vi "optionsAcq_channel_attenuatorState.vi"(6 "poll write":bool, 8 "error in (no error)":errorcluster, 9 "readWrite":enum16{"read", "write"}(ring), 10 "attenFilter_active":bool, 11 "OSAchannel in":refnum<class "OSAchannel.lvclass">) -> (0 "error out":errorcluster, 1 "FTSLib status":i32, 2 "attenFilter_active read":bool, 3 "OSAchannel out":refnum<class "OSAchannel.lvclass">, 4 "poll timeOut":bool)   [LabVIEW 2010, in "OSAchannel.lvclass"]
uses:
  OSAchannel.lvclass
  OSAchannel.lvclass/OSAchannel.ctl
  FTSLib.dll
  OSA20X_misc.lvlib
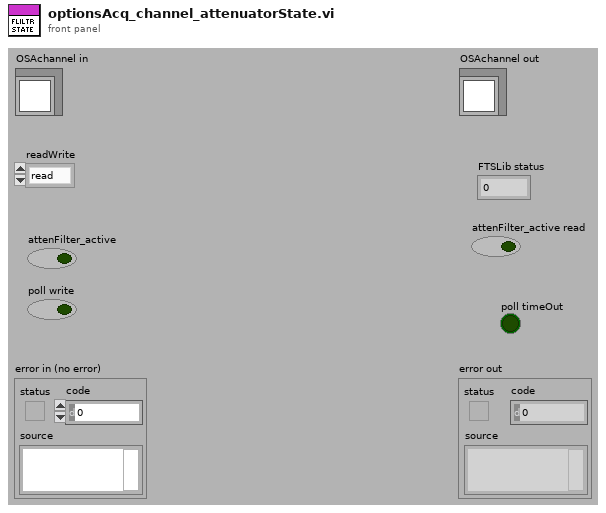
[diagram p1: front panel]
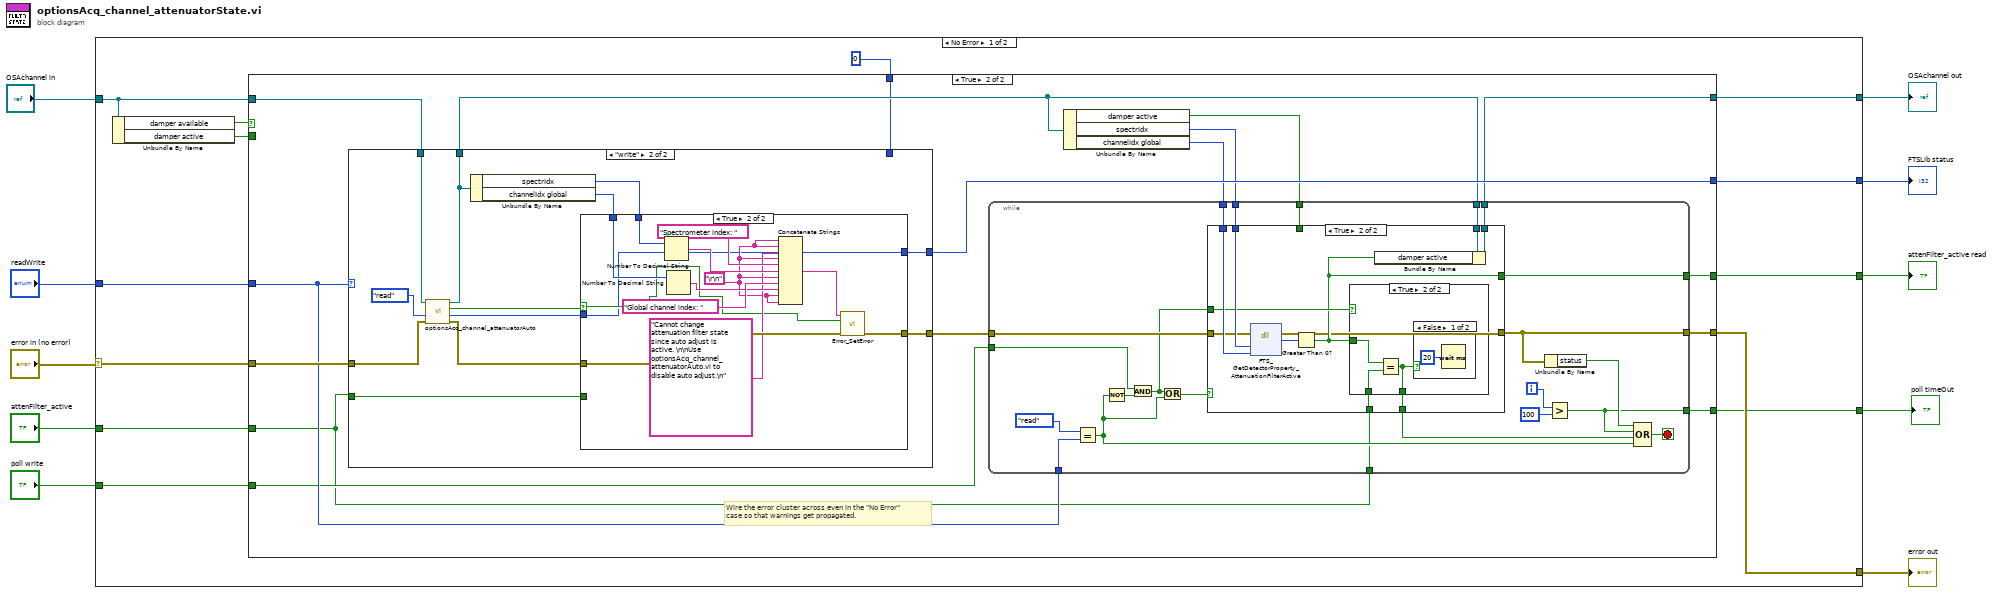
[diagram p0: block diagram]
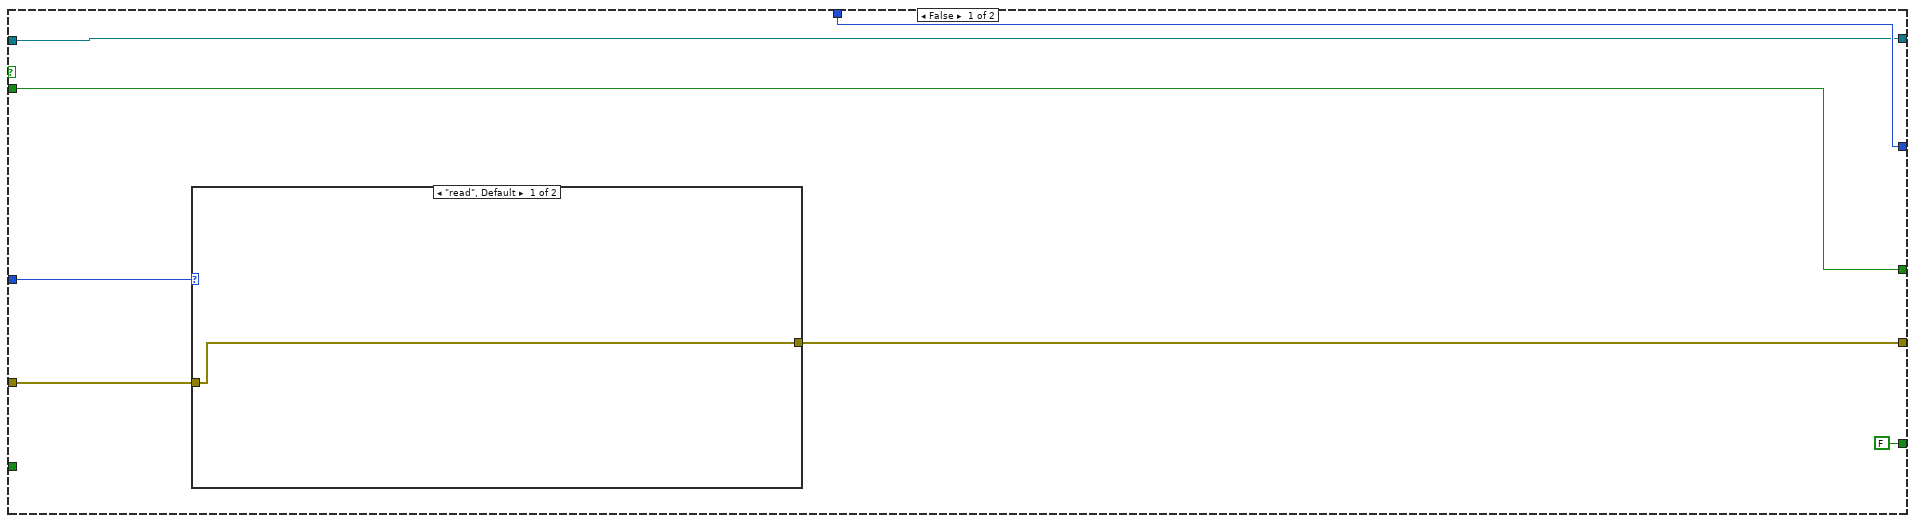
[diagram p2: hidden frame]
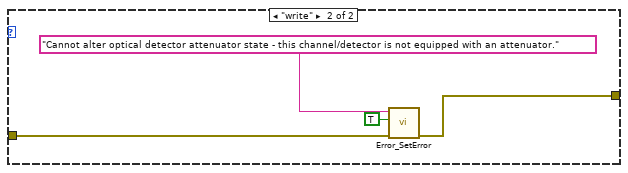
[diagram p3: hidden frame]
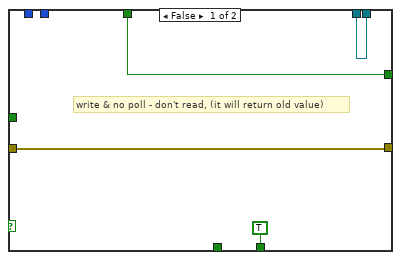
[diagram p4: hidden frame]
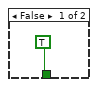
[diagram p5: hidden frame]
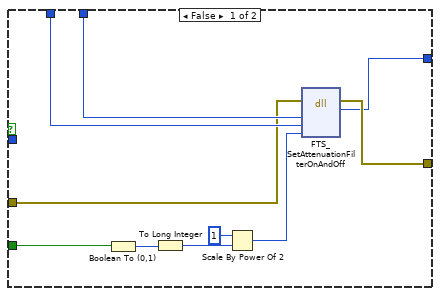
[diagram p8: hidden frame]
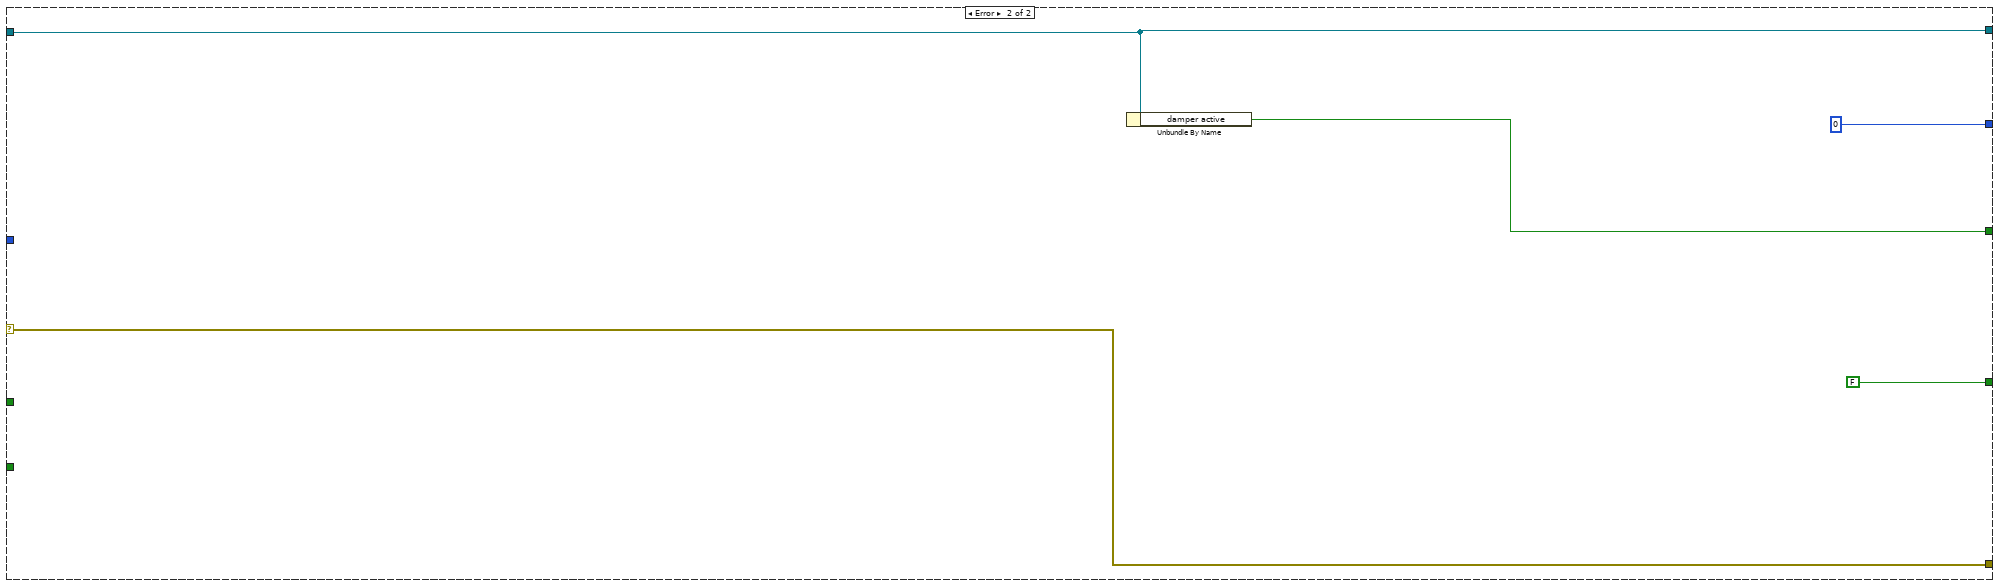
[diagram p9: hidden frame]
diagram:
  n1 = case shown="No Error" "error in (no error)" {
    selector: "error in (no error)" -> [w23 w136]
    tunnel: [w16 w136] -> w9
    tunnel: [w17 w135] -> w7
    tunnel: "OSAchannel in" -> [w14 w135]
    tunnel: "readWrite" -> [w21 _]
    tunnel: "attenFilter_active" -> [w19 _]
    tunnel: [w22 0 ("result")] -> w4
    tunnel: "poll write" -> [w20 _]
    tunnel: [w18 w134] -> w2
    tunnel: [w15 FALSE] -> w1
    frame No Error {
      n2 = Unbundle By Name(w14) -> ("damper available"=w13:bool, "damper active"=w12:bool)
      n3 = case shown="True" w13 {
        tunnel: w23 -> [w25 w51]
        tunnel: [w28 w50] -> w22
        tunnel: w21 -> [w26 w49]
        tunnel: w20 -> [_ w45]
        tunnel: w19 -> [_ w44]
        tunnel: [w30 w43] -> w18
        tunnel: [w27 w42] -> w17
        tunnel: [w24 w40] -> w16
        tunnel: [FALSE w39] -> w15
        tunnel: w14 -> [w27 w37]
        tunnel: w12 -> [w30 _]
        tunnel: 0 ("result") -> [w28 w36]
        frame False {
          n4 = case shown="\"read\", Default" w26 {
            tunnel: w25 -> [w31 w35]
            tunnel: [w31 w34] -> w24
            frame "read", Default {
            }
            frame "write" {
              n5 = call "Error_SetError.vi"("error in"=w35, "status (true)"=TRUE, "source(\"\")"="Cannot alter optical detector attenuator state - this channel/detector is not equipped with an attenuator." ("source(\"\")")) -> ("error out"=w34:errorcluster)  [unwired: 4 in]
            }
          }
        }
        frame True {
          # "Wire the error cluster across even in the \"No Error\"\ncase so that warnings get propagated."
          n6 = case shown="\"write\"" w49 {
            tunnel: [w96 w107] -> w50
            tunnel: w51 -> [w95 w99]
            tunnel: [w95 w108] -> w46
            tunnel: w44 -> [_ w106]
            tunnel: w36 -> [w96 _]
            tunnel: w37 -> [w94 w102]
            tunnel: [w94 w103] -> w38
            frame Default {
            }
            frame "write" {
              n7 = call "optionsAcq_channel_attenuatorAuto.vi"("error in (no error)"=w99, "readWrite"=enum16{"read", "write"}."read", "OSAchannel in"=w102) -> ("error out"=w98:errorcluster, "FTSLib status"=w97:i32, "auto read"=w101:bool, "OSAchannel out"=w103:refnum<class "OSAchannel.lvclass">)  [unwired: 5 in]
              n8 = Unbundle By Name(w103) -> ("spectrIdx"=w104:u16, "channelIdx global"=w105:u16)
              n9 = case shown="True" w101 {
                selector: w101 -> [_ w120]
                tunnel: w105 -> [w118 w128]
                tunnel: w104 -> [w117 w129]
                tunnel: w98 -> [w116 w131]
                tunnel: [w115 w130] -> w108
                tunnel: [w114 w119] -> w107
                tunnel: w106 -> [w109 _]
                tunnel: w97 -> [_ w119]
                frame False {
                  n10 = Boolean To (0,1)(Boolean=w109) -> (0, 1=w111:i16)
                  n11 = To Long Integer(number=w111) -> (32bit integer=w112:i32)
                  n12 = Scale By Power Of 2(n=1, x=w112) -> (x*2^n=w110:i32)
                  n13 = dll-call lib="FTSLib.dll" fn="FTS_SetAttenuationFilterOnAndOff"(error in=w116, "spectrIdx"=w117, "channeldx"=w118, "filterStatus"=w110) -> (error out=w115:errorcluster, "result"=w114:i32)  [unwired: 5 in, 1 out]
                }
                frame True {
                  w121 = "\r\n"
                  n14 = Number To Decimal String(number=w129) -> (decimal integer string=w126:string)  [unwired: 1 in]
                  n15 = Number To Decimal String(number=w128) -> (decimal integer string=w124:string)  [unwired: 1 in]
                  n16 = Concatenate Strings(w121, w121, "Cannot change attenuation filter state since auto adjust is active. \n\nUse optionsAcq_channel_attenuatorAuto.vi to disable auto adjust.\n" ("source(\"\")"), w121, "Spectrometer index: " ("string"), w126, w121, "Global channel index: " ("string"), w124, w121, w121) -> (w122:string)
                  n17 = call "Error_SetError.vi"("error in"=w131, "status (true)"=w120, "source(\"\")"=w122) -> ("error out"=w130:errorcluster)  [unwired: 4 in]
                }
              }
            }
          }
          n18 = Unbundle By Name(w38) -> ("damper active"=w41:bool, "spectrIdx"=w47:u16, "channelIdx global"=w48:u16)
          n19 = while {
            tunnel: w49 -> [w73]
            tunnel: w48 -> [w70]
            tunnel: w47 -> [w69]
            tunnel: w46 -> [w68]
            tunnel: w45 -> [w64]
            tunnel: w44 -> [w63]
            tunnel: [w60] -> w43
            tunnel: w38 -> [w59]
            tunnel: [w58] -> w42
            tunnel: w41 -> [w57]
            tunnel: [w53] -> w40
            tunnel: [w52] -> w39
            i -> [w56]
            stop <- w71 stop-if-true
            n20 = Equal?(x=enum16{"read", "write"}."read", y=w73) -> (x = y?=w67:bool)
            n21 = Not(x=w67) -> (.not. x?=w66:bool)
            n22 = And(x=w64, y=w66) -> (x .and. y?=w62:bool)
            n23 = Or(x=w62, y=w67) -> (x .or. y?=w65:bool)
            n24 = case shown="True" w65 {
              tunnel: w70 -> [_ w87]
              tunnel: w69 -> [_ w86]
              tunnel: w68 -> [w74 w85]
              tunnel: w63 -> [_ w84]
              tunnel: w62 -> [_ w83]
              tunnel: [TRUE w82] -> w61
              tunnel: [w75 w79] -> w60
              tunnel: w59 -> [w76 w81]
              tunnel: [w76 w80] -> w58
              tunnel: w57 -> [w75 _]
              tunnel: [w74 w78] -> w53
              frame False {
                # "write & no poll - don't read, (it will return old value)"
              }
              frame True {
                n25 = dll-call lib="FTSLib.dll" fn="FTS_GetDetectorProperty_AttenuationFilterActive"(error in=w85, "spectrIdx"=w86, "channeldx"=w87) -> (error out=w78:errorcluster, "attenuatorActive"=w88:i32)  [unwired: 4 in, 1 out]
                n26 = Greater Than 0?(x=w88) -> (x > 0?=w79:bool)
                n27 = case shown="True" w83 {
                  tunnel: w79 -> [_ w91]
                  tunnel: w84 -> [_ w92]
                  tunnel: [TRUE w90] -> w82
                  frame False {
                  }
                  frame True {
                    n28 = Equal?(x=w91, y=w92) -> (x = y?=w90:bool)
                    n29 = case shown="False" w90 {
                      frame False {
                        n30 = Wait (ms)(milliseconds to wait=u32 20) -> ()  [unwired: 1 out]
                      }
                      frame True {
                      }
                    }
                  }
                }
                n31 = Bundle By Name(cluster=w81, "damper active"=w79) -> (w80:refnum<class "OSAchannel.lvclass">)
              }
            }
            n32 = Unbundle By Name(w53) -> ("status"=w54:bool)
            n33 = Greater?(x=w56, y=100) -> (0:w52:bool)
            n34 = Compound Arithmetic op=OR(w54, w52, w61, w67) -> (w71:bool)
          }
        }
      }
    }
    frame Error {
      n35 = Unbundle By Name(w135) -> ("damper active"=w134:bool)
    }
  }
  "error out" <- w9
  "OSAchannel out" <- w7
  "attenFilter_active read" <- w2
  "FTSLib status" <- w4
  "poll timeOut" <- w1
